vi "flicker test with zero4.vi"() -> ()   [LabVIEW 2013]
uses:
  <instrlib>/Tektronix DPO MSO 2000 4000 Series/Public/Data/Data_Low Level/Fetch Waveform (Waveform Data Type).vi
  <instrlib>/Tektronix DPO MSO 2000 4000 Series/Tektronix DPO MSO 2000 4000 Series.lvlib
panel:
  in  "Notes (plain text, no commas)":string
  in  "Amp gain":string
  in  "Test repeat #":string
  in  "Dim level% (3 sig fig)\n\"100\" if no dimming)":string
  in  "Dimmer descriptoin\n(\"power supply\" for no\ndimming also)":string
  in  "Model (eg. \"omni05\")":string
  in  "Maximum Time (10000ms)":u32=10000
  in  "VISA Resource Name":refnum<visa-resource-name>
  out "appended path":path
  out "data":waveform(dbl)(graph)
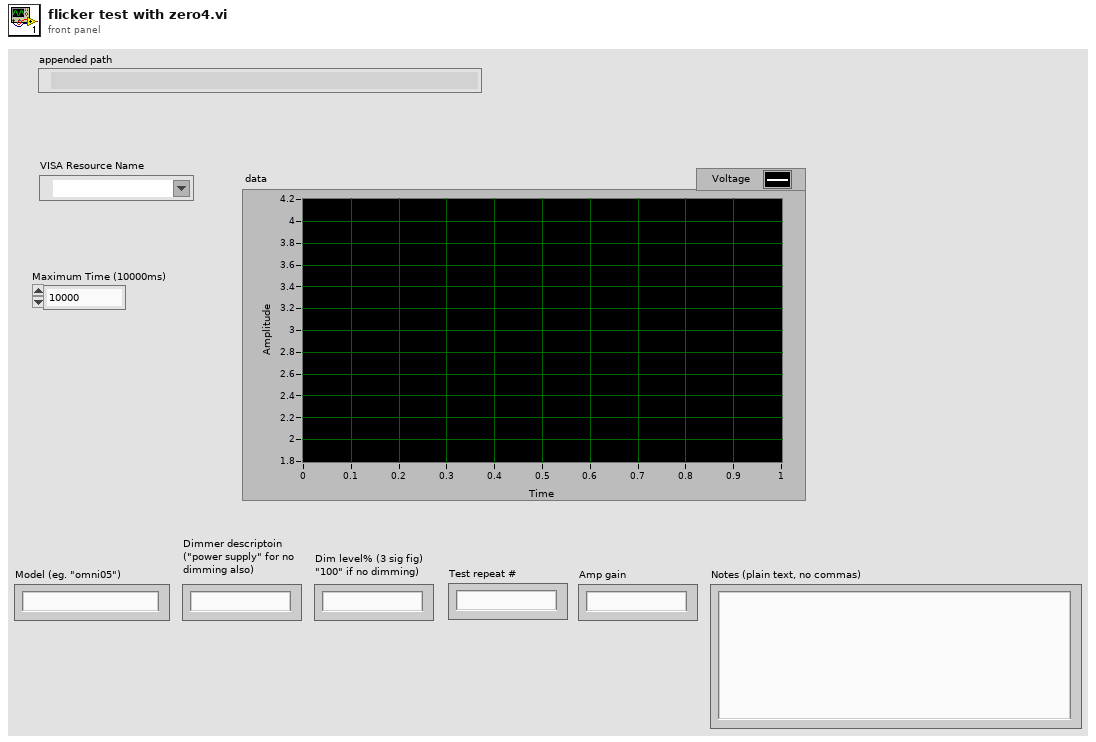
[diagram p1: front panel]
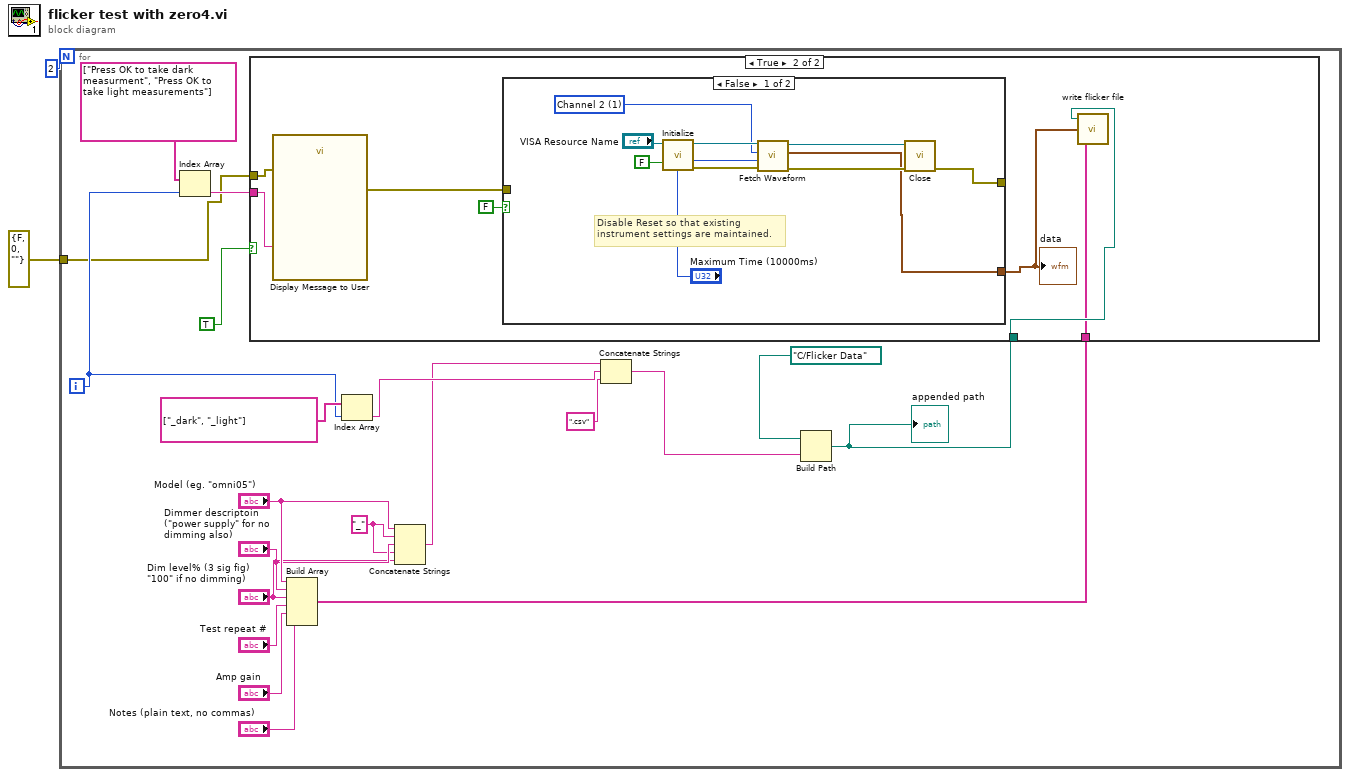
[diagram p0: block diagram]
diagram:
  n1 = for {
    N: 2 -> [_]
    tunnel: errorcluster {"status"=FALSE, "code"=0, "source"=""} ("error constant") -> [w3]
    i -> [w17]
    w9 = "_"
    n2 = Index Array(array=string[] ["Press OK to take dark measurment", "Press OK to take light measurements"], index=w17) -> (element=w21:string)
    n3 = Build Array("Model (eg. \"omni05\")", "Dimmer descriptoin\n(\"power supply\" for no\ndimming also)", "Dim level% (3 sig fig)\n\"100\" if no dimming)", "Test repeat #", "Amp gain", "Notes (plain text, no commas)") -> (w6:string[])
    n4 = Index Array(array=string[] ["_dark", "_light"], index=w17) -> (element=w15:string)
    n5 = Concatenate Strings("Model (eg. \"omni05\")", w9, "Dimmer descriptoin\n(\"power supply\" for no\ndimming also)", w9, "Dim level% (3 sig fig)\n\"100\" if no dimming)") -> (w7:string)
    n6 = Concatenate Strings(w7, w15, ".csv" ("string")) -> (w20:string)
    n7 = Build Path(base path=path "C:/Flicker Data", name or relative path=w20) -> (appended path=w19:path)
    "appended path" <- w19
    n8 = case shown="True" TRUE {
      tunnel: w21 -> [_ w28]
      tunnel: w19 -> [_ w27]
      tunnel: w6 -> [_ w26]
      tunnel: w3 -> [_ w25]
      frame False {
      }
      frame True {
        n9 = call "Display Message to User"("error in (no error)"=w25, "Message"=w28) -> ("error out"=w29:errorcluster)  [unwired: 8 in, 1 out]
        n10 = case shown="False" FALSE {
          tunnel: w29 -> [_ w40]
          tunnel: [w31 w40] -> _
          tunnel: [w30 _] -> w23
          frame False {
            w33 = u16 1 items=["Channel 1", "Channel 2", "Channel 3", "Channel 4", "Math", "Reference 1", "Reference 2", "Reference 3", "Reference 4", "D0", "D1", "D2", "D3", "D4", "D5", "D6", "D7", "D8", "D9", "D10", "D11", "D12", "D13", "D14", "D15", "Amplitude", "Frequency", "Phase", "Normal", "Average", "Maximum Peak Hold", "Minimum Peak Hold"] ("Channel (0: Channel 1)")
            # "Disable Reset so that existing\ninstrument settings are maintained."
            n11 = call <instrlib>:"Initialize.vi"("Reset (True)"=FALSE ("Reset? (T: Yes)"), "VISA resource name"="VISA Resource Name") -> ("error out"=w36:errorcluster, "VISA resource name out"=w37:refnum<visa-resource-name>)  [unwired: 8 in]
            n12 = call-poly <instrlib>:"Fetch Waveform.vi"("error in (no error)"=w36, "Maximum Time (10000ms)"="Maximum Time (10000ms)", "Channel (0: Channel 1)"=w33, "VISA resource name"=w37) -> ("error out"=w35:errorcluster, "Waveform Data"=w30:waveform(dbl), "VISA resource name out"=w32:refnum<visa-resource-name>)  [unwired: 5 in]
            n13 = call <instrlib>:"Close.vi"("error in (no error)"=w35, "VISA resource name"=w32) -> ("error out"=w31:errorcluster)  [unwired: 9 in]
          }
          frame True {
          }
        }
        "data" <- w23
        n14 = call "write flicker file.vi"("Array"=w26, "Waveform Data"=w23, "appended path"=w27) -> ()  [unwired: 1 in]
      }
    }
  }
